vi "IVIS FRET_Load Image as SGL.vi"(8 "error in":errorcluster, 10 "Image File Name":string, 11 "Root Folder":path) -> (0 "error out":errorcluster, 1 "Y Resolution":i32, 2 "X Resolution":i32, 3 "Background Image":T1)   [LabVIEW 2021]
uses:
  <vilib>/vision/Image Controls.llb/IMAQ Image.ctl
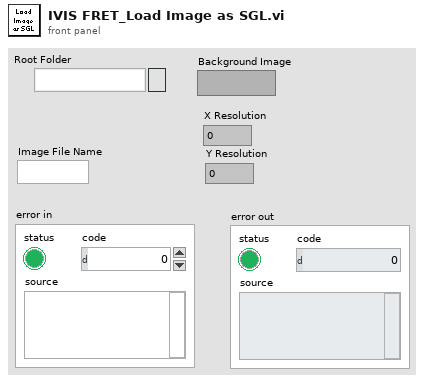
[diagram p1: front panel]
types:
  T1 = typedef "IMAQ Image.ctl" = refnum<image>
  T2 = typedef "Image Type" = u32
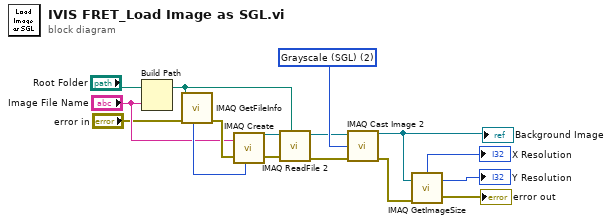
[diagram p0: block diagram]
diagram:
  w16 = T2 2 items=["Grayscale (U8)", "Grayscale (I16)", "Grayscale (SGL)", "Complex (CSG)", "RGB (U32)", "HSL (U32)", "RGB (U64)", "Grayscale (U16)"] ("Image Type")
  n1 = Build Path(base path="Root Folder", name or relative path="Image File Name") -> (appended path=w11:path)
  n2 = call "IMAQ GetFileInfo"("error in (no error)"="error in", "File Path"=w11) -> ("error out"=w9:errorcluster, "Image Type"=w8:T2)  [unwired: 3 in, 5 out]
  n3 = call "IMAQ Create"("Image Name"="Image File Name", "Image Type"=w8, "error in (no error)"=w9) -> ("New Image"=w12:T1, "error out"=w10:errorcluster)  [unwired: 2 in]
  n4 = call "IMAQ ReadFile 2"("File Path"=w11, "error in (no error)"=w10, "Image"=w12) -> ("error out"=w15:errorcluster, "Image Out"=w14:T1)  [unwired: 4 in, 3 out]
  n5 = call "IMAQ Cast Image 2"("Image Src"=w14, "Image Type"=w16, "error in (no error)"=w15) -> ("Image Dst Out"=w1:T1, "error out"=w5:errorcluster)  [unwired: 11 in]
  "Background Image" <- w1
  n6 = call "IMAQ GetImageSize"("Image"=w1, "error in (no error)"=w5) -> ("Y Resolution"=→"Y Resolution":i32, "X Resolution"=→"X Resolution":i32, "error out"=→"error out":errorcluster)  [unwired: 2 in]
